vi "Set Hierarchy Root.vi"(8 "error in (no error)":errorcluster, 10 "Hierarchy Root":string[](array[string]), 11 "Pref Group in":refnum<class "Pref Group.lvclass">) -> (0 "error out":errorcluster, 3 "Pref Group out":refnum<class "Pref Group.lvclass">)   [LabVIEW 2020, in "User Prefs.lvlib" / "Pref Group.lvclass"]
uses:
  Pref Group.lvclass
  Pref Group.lvclass/Pref Group.ctl
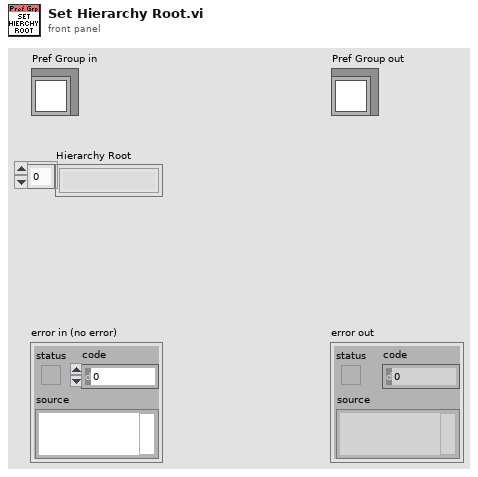
[diagram p1: front panel]
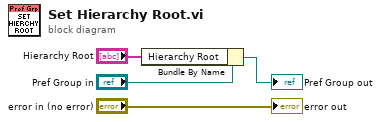
[diagram p0: block diagram]
diagram:
  n1 = Bundle By Name(cluster="Pref Group in", "Hierarchy Root"="Hierarchy Root") -> (→"Pref Group out":refnum<class "Pref Group.lvclass">)
  "error out" <- "error in (no error)"
